vi "401_Customized_Data.vi"(8 "error in":errorcluster, 9 "End_date":string, 10 "Start_date":string, 11 "connection in":T1) -> (0 "error Out":errorcluster, 2 "Data_Table":string[][](array[string]), 3 "connection out":T1)   [LabVIEW 2015]
uses:
  <vilib>/addons/database/Connection.llb/Conn ObjectReference.ctl
  <vilib>/addons/database/NI_Database_API.lvlib
panel:
  # "Input"
  # "Output"
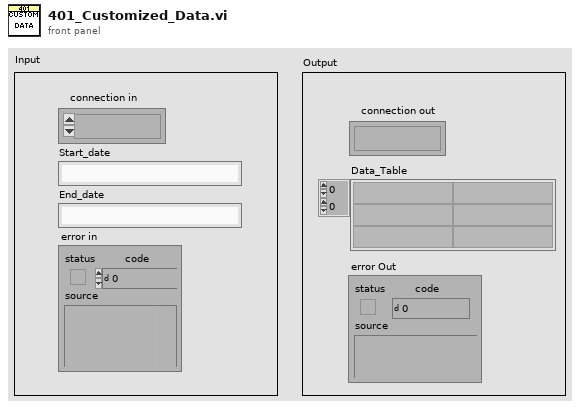
[diagram p1: front panel]
types:
  T1 = typedef "NI_Database_API.lvlib/Conn ObjectReference.ctl" = refnum<k1>
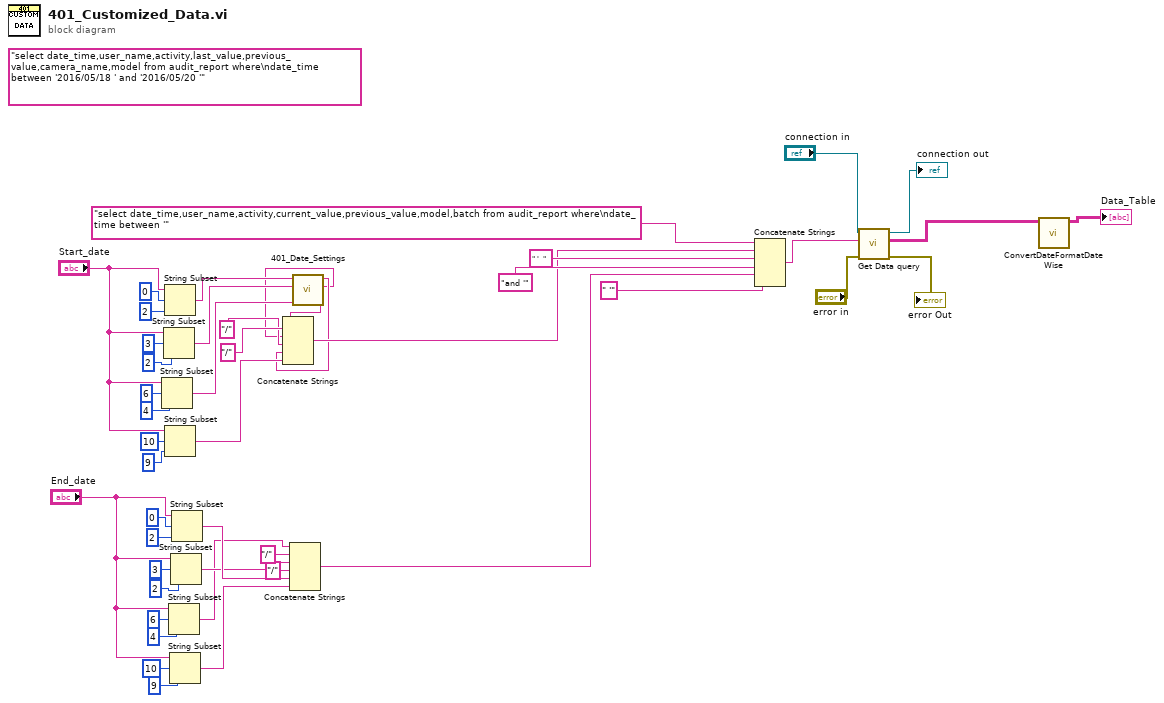
[diagram p0: block diagram]
diagram:
  (unwired) "select date_time,user_name,activity,last_value,previous_value,camera_name,model from audit_report where\ndate_time between '2016/05/18 ' and '2016/05/20 '" ("SQL query")
  n1 = String Subset(string="Start_date", offset (0)=6, length (rest)=4 ("length (rest)")) -> (substring=w5:string)
  n2 = String Subset(string="Start_date", offset (0)=3, length (rest)=2 ("length (rest)")) -> (substring=w6:string)
  n3 = String Subset(string="Start_date", offset (0)=0, length (rest)=2 ("length (rest)")) -> (substring=w7:string)
  n4 = String Subset(string="Start_date", offset (0)=10, length (rest)=9 ("length (rest)")) -> (substring=w9:string)
  n5 = String Subset(string="End_date", offset (0)=6, length (rest)=4 ("length (rest)")) -> (substring=w13:string)
  n6 = String Subset(string="End_date", offset (0)=10, length (rest)=9 ("length (rest)")) -> (substring=w11:string)
  n7 = String Subset(string="End_date", offset (0)=3, length (rest)=2 ("length (rest)")) -> (substring=w31:string)
  n8 = String Subset(string="End_date", offset (0)=0, length (rest)=2 ("length (rest)")) -> (substring=w33:string)
  n9 = Concatenate Strings(w13, "/" ("string"), w31, "/" ("string"), w33, w11) -> (w19:string)
  n10 = call "401_Date_Settings.vi"("Year"=w5, "Month"=w6, "Start_date"=w7) -> ("Year"=w4:string, "Month"=w3:string, "Date"=w8:string)  [unwired: 6 in]
  n11 = Concatenate Strings(w4, "/" ("string"), w3, "/" ("string"), w8, w9) -> (w36:string)
  n12 = Concatenate Strings("select date_time,user_name,activity,current_value,previous_value,model,batch from audit_report where\ndate_time between '" ("string"), w36, " '  " ("string"), "and '" ("string"), w19, " '" ("string")) -> (w10:string)
  n13 = call "Get Data query.vi"("error in"="error in", "SQL query"=w10, "connection reference"="connection in") -> ("error Out"=→"error Out":errorcluster, "Data_Table"=w2:string[][], "connection reference"=→"connection out":T1)  [unwired: 6 in]
  n14 = call "ConvertDateFormatDateWise.vi"("DataIn"=w2) -> ("DataOut"=→"Data_Table":string[][])  [unwired: 10 in]
